vi "Set Data Type.vi"(8 "error in (no error)":errorcluster, 9 "Data Type":enum16{"Voltage", "Raw"}(ring), 11 "VISA resource name":refnum<visa-resource-name>) -> (0 "error out":errorcluster, 3 "VISA resource name out":refnum<visa-resource-name>)   [LabVIEW 2020, in "BDAQ-6104.lvlib"]
doc: "Set the analog output data type. Voltage or raw DAC data."
uses:
  <instrlib>/BDAQ-6104/BDAQ-6104.lvlib
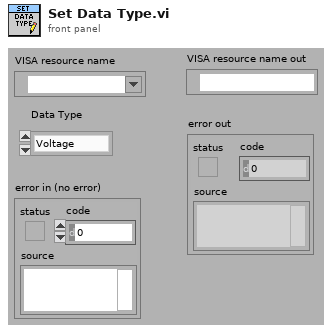
[diagram p1: front panel]
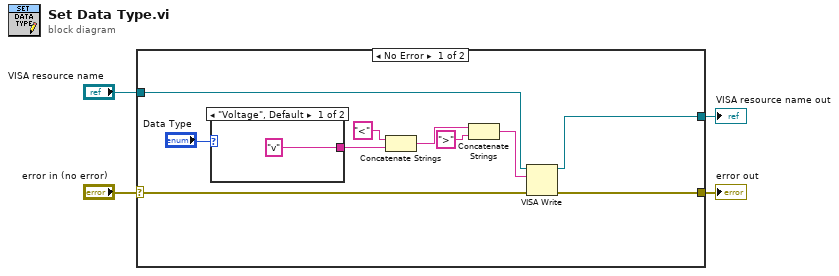
[diagram p0: block diagram]
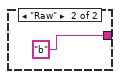
[diagram p2: hidden frame]
diagram:
  n1 = case shown="No Error" "error in (no error)" {
    selector: "error in (no error)" -> [w7 w18]
    tunnel: [w13 w18] -> w4
    tunnel: "VISA resource name" -> [w6 w17]
    tunnel: [w5 w17] -> w1
    frame No Error {
      n2 = case shown="\"Voltage\", Default" "Data Type" {
        tunnel: ["v" "b"] -> w8
        frame "Voltage", Default {
        }
        frame "Raw" {
        }
      }
      n3 = Concatenate Strings("<" ("command"), w8) -> (w11:string)
      n4 = Concatenate Strings(w11, ">" ("command")) -> (w12:string)
      n5 = VISA Write(VISA resource name=w6, write buffer=w12, error in (no error)=w7) -> (VISA resource name out=w5:refnum<visa-resource-name>, error out=w13:errorcluster)  [unwired: 1 out]
    }
    frame Error {
    }
  }
  "error out" <- w4
  "VISA resource name out" <- w1
